vi "Pose Update Queue Loop.vi"() -> (3 "Estimated Pose (Degrees)":cluster{"X":dbl, "Y":dbl, "R":dbl})   [LabVIEW 2018]
uses:
  Control Globals.vi
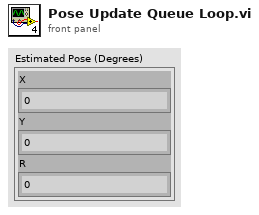
[diagram p1: front panel]
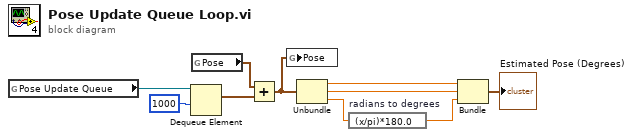
[diagram p0: block diagram]
diagram:
  n1 = global read "Control Globals.vi" "Pose Update Queue"() -> (w1:refnum<queue>)
  n2 = Dequeue Element(queue=w1, timeout in ms (-1)=1000) -> (element=w9:cluster{"X":dbl, "Y":dbl, "R":dbl})  [unwired: 1 in, 3 out]
  n3 = global read "Control Globals.vi" "Pose"() -> (w3:cluster{"X":dbl, "Y":dbl, "R":dbl})
  n4 = Add(x=w3, y=w9) -> (x+y=w2:cluster{"X":dbl, "Y":dbl, "R":dbl})
  n5 = global write "Control Globals.vi" "Pose"(w2) -> ()
  n6 = Unbundle(w2) -> ("X"=w8:dbl, "Y"=w7:dbl, "R"=w6:dbl)
  n7 = expression code="(x/pi)*180.0" "radians to degrees"(w6) -> (w5:dbl)
  n8 = Bundle("X"=w8, "Y"=w7, "R"=w5) -> (→"Estimated Pose (Degrees)":cluster{"X":dbl, "Y":dbl, "R":dbl})  [unwired: 1 in]
